vi "Send Value to Excel.vi"(11 "Value":string="SendKeys %fn") -> (0 "error out":errorcluster)   [LabVIEW 2012]
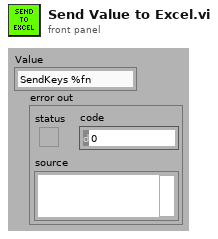
[diagram p1: front panel]
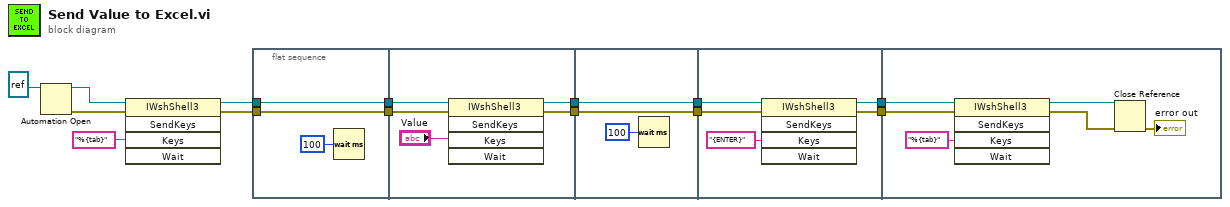
[diagram p0: block diagram]
diagram:
  n1 = Automation Open(Automation Refnum=refnum<k7> refnum ("IWshRuntimeLibrary.IWshShell3")) -> (Automation Refnum=w12:refnum<k7>, error out=w13:errorcluster)  [unwired: 3 in]
  n2 = invoke class="IWshShell3" method="SendKeys"(reference=w12, error in=w13, "Keys"="%{tab}") -> (reference out=w11:refnum<k7>, error out=w10:errorcluster)  [unwired: 2 in, 3 out]
  n3 = flat-sequence {
    tunnel: w10 -> [w16]
    tunnel: w11 -> [w17]
    tunnel: [w17] -> w8
    tunnel: [w16] -> w7
    tunnel: w8 -> [w22]
    tunnel: w7 -> [w21]
    tunnel: [w19] -> w5
    tunnel: [w18] -> w4
    tunnel: [w24] -> w6
    tunnel: w5 -> [w24]
    tunnel: w4 -> [w23]
    tunnel: [w23] -> w3
    tunnel: w6 -> [w29]
    tunnel: w3 -> [w28]
    tunnel: [w27] -> w2
    tunnel: [w26] -> w1
    tunnel: w2 -> [w33]
    tunnel: w1 -> [w32]
    frame #0 {
      n4 = Wait (ms)(milliseconds to wait=u32 100) -> ()  [unwired: 1 out]
    }
    frame #1 {
      n5 = invoke class="IWshShell3" method="SendKeys"(reference=w22, error in=w21, "Keys"="Value") -> (reference out=w19:refnum<k7>, error out=w18:errorcluster)  [unwired: 2 in, 3 out]
    }
    frame #2 {
      n6 = Wait (ms)(milliseconds to wait=u32 100) -> ()  [unwired: 1 out]
    }
    frame #3 {
      n7 = invoke class="IWshShell3" method="SendKeys"(reference=w29, error in=w28, "Keys"="{ENTER}" ("Keys 3")) -> (reference out=w27:refnum<k7>, error out=w26:errorcluster)  [unwired: 2 in, 3 out]
    }
    frame #4 {
      n8 = invoke class="IWshShell3" method="SendKeys"(reference=w33, error in=w32, "Keys"="%{tab}" ("Keys 3")) -> (reference out=w36:refnum<k7>, error out=w34:errorcluster)  [unwired: 2 in, 3 out]
      n9 = Close Reference(reference=w36, error in (no error)=w34) -> (error out=→"error out":errorcluster)
    }
  }
